vi "make1And2.vi"(6 "emptyZArrayforreshape in":T5, 9 "X size":dbl, 10 "CamSettings":T1={"Cam 0"={"position"=0.0, "Field of view"=0.0, "start"=0.0, "end"=0.0, "center"=0.0, "Lens"=enum."FL1-f8x08", "Forward"=enum."off", "Spec_Calib_file 2"=path "Y:/100TWdata/ESMCalib/datFwd.txt", "map"=path "Y:/100TWdata/ESMCalib/mapFwd.txt", "y size"=0}, "Cam 1"={"position"=0.0, "Field of view"=0.0, "start"=0.0, "end"=0.0, "center"=0.0, "Lens"=enum."FL1-f8x08", "Forward"=enum."off", "Spec_Calib_file 2"=path "Y:/100TWdata/ESMCalib/datFwd.txt", "map"=path "Y:/100TWdata/ESMCalib/mapFwd.txt", "y size"=0}, "Cam 2"={"position"=0.0, "Field of view"=0.0, "start"=0.0, "end"=0.0, "center"=0.0, "Lens"=enum."FL1-f8x08", "Forward"=enum."off", "Spec_Calib_file 2"=path "Y:/100TWdata/ESMCalib/datFwd.txt", "map"=path "Y:/100TWdata/ESMCalib/mapFwd.txt", "y size"=0}, "Cam 3"={"position"=0.0, "Field of view"=0.0, "start"=0.0, "end"=0.0, "center"=0.0, "Lens"=enum."FL1-f8x08", "Forward"=enum."off", "Spec_Calib_file 2"=path "Y:/100TWdata/ESMCalib/datFwd.txt", "map"=path "Y:/100TWdata/ESMCalib/mapFwd.txt", "y size"=0}}, 11 "MaxY":i32) -> (2 "emptyZArrayforreshape out":T5, 3 "min Y":i32)   [LabVIEW 2011, in "MagAnalysis_Online.lvclass"]
uses:
  MagAnalysis_Online.lvclass
  emptyArray_TYpDEf.ctl
  emptyArrayCamX_TypDef.ctl
  CamSettings_Typdef.ctl
  CamSettingSUB_TypDEf.ctl
  CamAndObj_TypDEf.ctl
  OnOffTypeDef.ctl
panel:
  out "size(s) 2":i32[](array[numeric])
  out "size(s)":i32[](array[numeric])
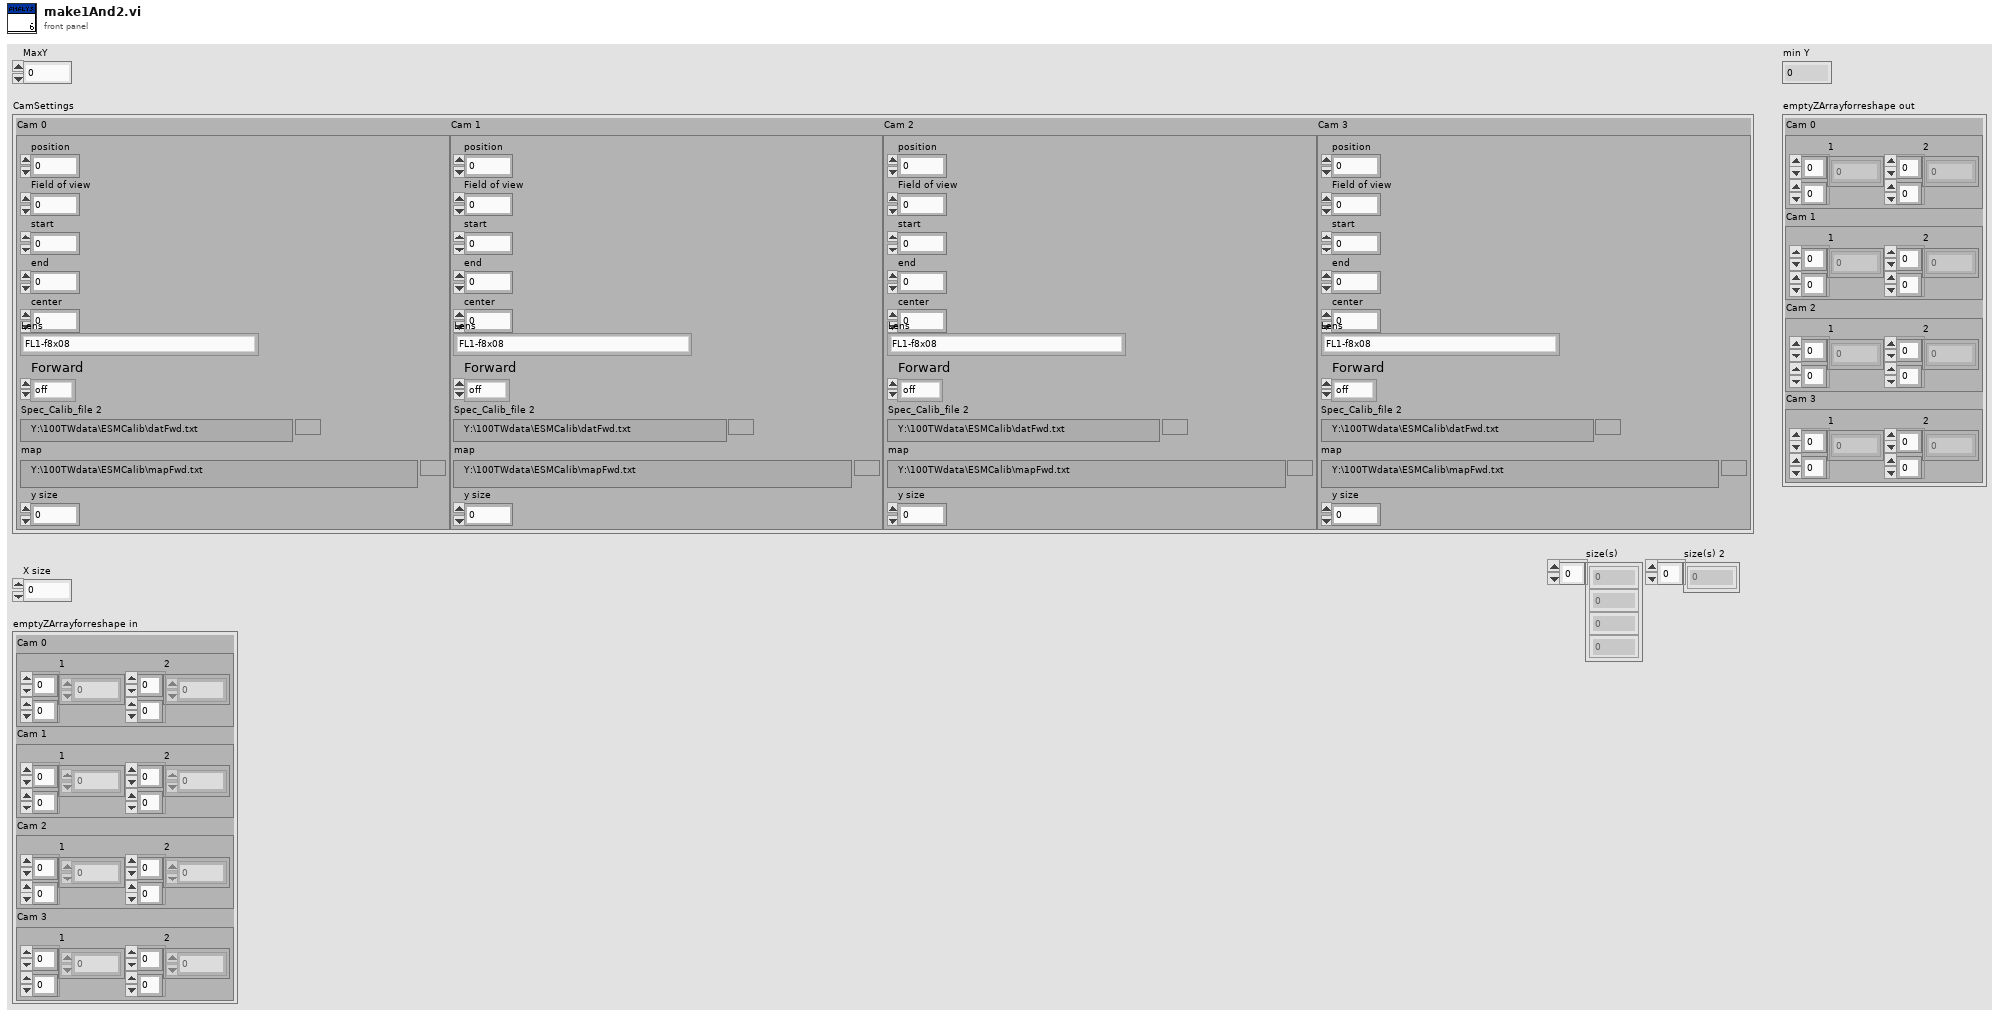
[diagram p1: front panel]
types:
  T1 = typedef "CamSettings_Typdef.ctl" = cluster{"Cam 0":T2, "Cam 1":T2, "Cam 2":T2, "Cam 3":T2}
  T2 = typedef "CamSettingSUB_TypDEf.ctl" = cluster{"position":dbl, "Field of view":dbl, "start":dbl, "end":dbl, "center":dbl, "Lens":T3, "Forward":T4, "Spec_Calib_file 2":path, "map":path, "y size":i32}
  T3 = typedef "CamAndObj_TypDEf.ctl" = enum16{"FL1-f8x08", "FL1-f8x06", "FL1-f8", "ch300-f50", "FL2G-f8", "FL3M14-f8", "FL3M14-f8x08", "FL3M14-f8x08(2x2)"}
  T4 = typedef "OnOffTypeDef.ctl" = enum16{"off", "on"}
  T5 = typedef "emptyArray_TYpDEf.ctl" = cluster{"Cam 0":T6, "Cam 1":T6, "Cam 2":T6, "Cam 3":T6}
  T6 = typedef "emptyArrayCamX_TypDef.ctl" = cluster{"1":dbl[][], "2":dbl[][]}
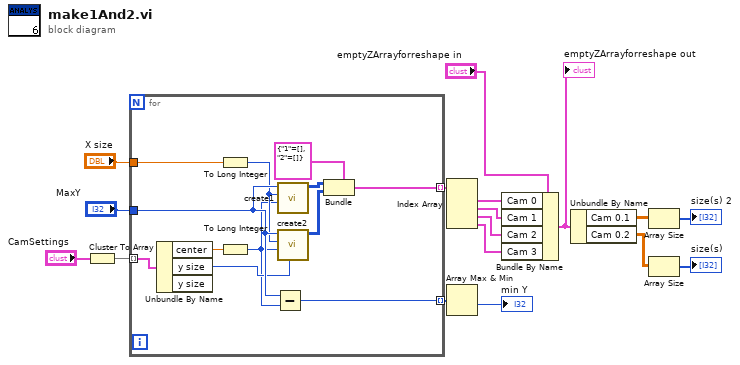
[diagram p0: block diagram]
diagram:
  n1 = Cluster To Array(cluster="CamSettings") -> (array=w13:T2[])
  n2 = for {
    tunnel: w13 -> [w29] mode=indexing
    tunnel: "MaxY" -> [w27]
    tunnel: [w28] -> w12 mode=indexing
    tunnel: "X size" -> [w25]
    tunnel: [w18] -> w11 mode=indexing
    n3 = Unbundle By Name(w29) -> ("center"=w23:dbl, "y size"=w26:i32)  [unwired: 1 out]
    n4 = To Long Integer(number=w25) -> (32bit integer=w24:i32)
    n5 = To Long Integer(number=w23) -> (32bit integer=w22:i32)
    n6 = Subtract(x=w27, y=w22) -> (x-y=w28:i32)
    n7 = call "create1.vi"("center"=w22, "X size"=w24, "max Y size"=w27) -> ("Array"=w21:i32[][])  [unwired: 7 in, 1 out]
    n8 = call "create2.vi"("actual y size"=w26, "center"=w22, "X size"=w24, "max Y size"=w27) -> ("Array"=w20:i32[][])  [unwired: 6 in, 1 out]
    n9 = Bundle(cluster=T6 {"1"=[], "2"=[]} ("Cam 1"), "1"=w21, "2"=w20) -> (w18:T6)
  }
  n10 = Index Array(array=w11) -> (element #1=w9:T6, element #2=w8:T6, element #3=w7:T6, element #4=w6:T6)  [unwired: 4 in]
  n11 = Array Max & Min(array=w12) -> (min value=→"min Y":i32)  [unwired: 3 out]
  n12 = Bundle By Name(cluster="emptyZArrayforreshape in", "Cam 0"=w9, "Cam 1"=w8, "Cam 2"=w7, "Cam 3"=w6) -> (w5:T5)
  "emptyZArrayforreshape out" <- w5
  n13 = Unbundle By Name(w5) -> ("Cam 0.1"=w4:dbl[][], "Cam 0.2"=w3:dbl[][])
  n14 = Array Size(array=w4) -> (size(s)=→"size(s) 2":i32[])
  n15 = Array Size(array=w3) -> (size(s)=→"size(s)":i32[])
